vi "Get Path to Plugin UI.vi"(8 "error in (no error)":errorcluster, 11 "Plugin Info":T1 {"Node Status"."Monitor Doubles"."4" format="%#_9g"; "Node Status"."Monitor Doubles"."3" format="%#_9g"; "Node Status"."Monitor Doubles"."2" format="%#_9g"; "Node Status"."Monitor Doubles"."1" format="%#_9g"; "Node Status"."Timing Statistics (us)"."Period"."Avg" format="%_6g"}) -> (0 "error out":errorcluster, 3 "Plugin UI Path":path)   [LabVIEW 2021, in "CIF_Manager_UI.lvclass"]
uses:
  CIF_Manager_UI.lvclass
  Typedef/PluginInfo.ctl
  <vilib>/CIF Foundation/CIF Core/CIFCore/Common/Typedef/Version Simple.ctl
  <vilib>/CIF Foundation/CIF Core/CIFCore/Common/Typedef/gRPC Reported Plugin Status.ctl
  <vilib>/CIF Foundation/CIF Core/CIFCore/Common/Typedef/Plugin State.ctl
  <vilib>/CIF Foundation/CIF Core/CIFCore/Common/Typedef/Timing Statistics.ctl
  <vilib>/CIF Foundation/CIF Core/CIFCore/Common/Typedef/Timing Stats Base.ctl
  <vilib>/CIF Foundation/CIF Core/CIFCore/Common/Typedef/FIFO Statistics.ctl
  <vilib>/CIF Foundation/CIF Core/CIFCore/Common/Typedef/Simple Error.ctl
  <vilib>/CIF Foundation/CIF Core/CIFCore/Common/Typedef/Monitor Doubles.ctl
  <vilib>/CIF Foundation/CIF Core/CIFCore/Common/Typedef/Monitor U64.ctl
  <vilib>/CIF Foundation/CIF Core/CIFCore/Common/Typedef/Monitor I64.ctl
  <vilib>/CIF Foundation/CIF Core/CIFUtilities/CIFConfigurationFile/typedef/Location Type.ctl
  <vilib>/CIF Foundation/CIF Core/CIFCore/Common/Typedef/Errors.ctl
  <vilib>/CIF Foundation/CIF Utilities/Errors/Append Error Location.vi
  <vilib>/CIF Foundation/CIF Core/CIFUtilities/CIFConfigurationFile/CIF Configuration File Location.vi
  <vilib>/CIF Foundation/CIF Core/CIFCore/Common/CIFCoreCommon.lvlib
  <vilib>/CIF Foundation/CIF Core/CIFUtilities/CIFConfigurationFile/CIF Configuration File.lvlib
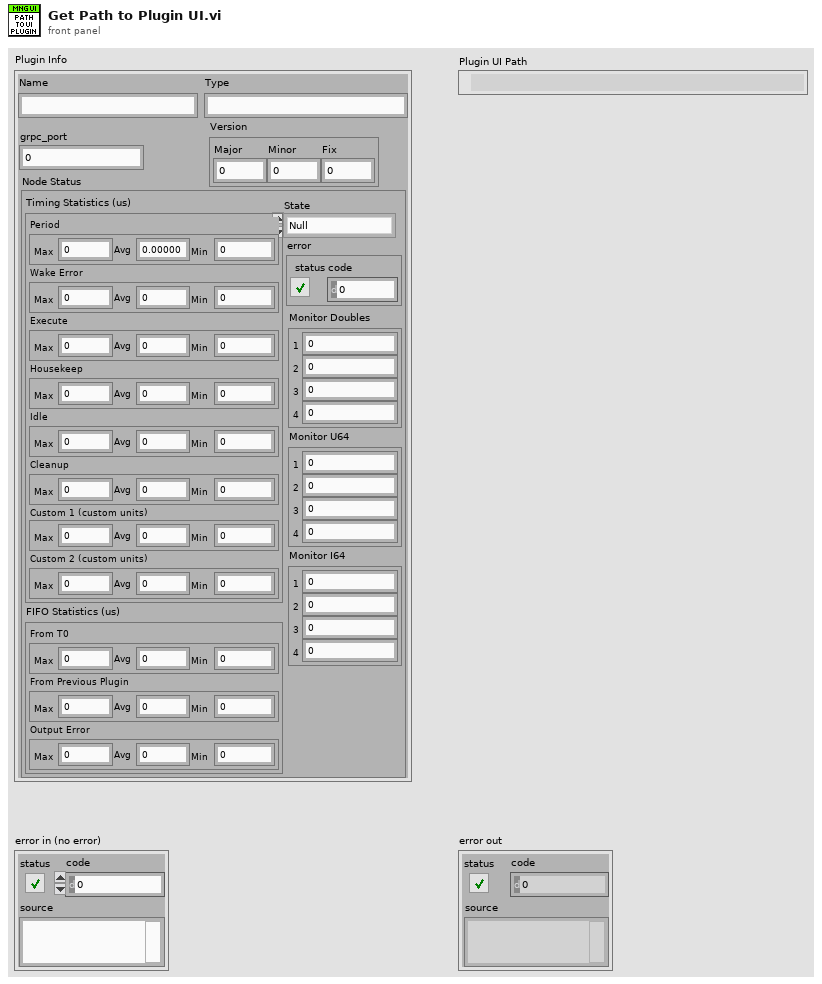
[diagram p1: front panel]
types:
  T1 = typedef "CIF_Manager_UI.lvclass/PluginInfo.ctl" = cluster{"Name":string, "Type":string, "grpc_port":i32, "Version":T2, "Node Status":T3}
  T2 = typedef "CIFCoreCommon.lvlib/Version Simple.ctl" = cluster{"Major":i32, "Minor":i32, "Fix":i32}
  T3 = typedef "CIFCoreCommon.lvlib/gRPC Reported Plugin Status.ctl" = cluster{"State":T4, "Timing Statistics (us)":T5, "FIFO Statistics (us)":T7, "error":T8, "Monitor Doubles":T9, "Monitor U64":T10, "Monitor I64":T11}
  T4 = typedef "CIFCoreCommon.lvlib/Plugin State.ctl" = enum32{"Null", "Creating", "Listening", "Running", "CleaningUp", "Destroying", "Prepared", "FTE_Run"}
  T5 = typedef "CIFCoreCommon.lvlib/Timing Statistics.ctl" = cluster{"Period":T6, "Wake Error":T6, "Execute":T6, "Housekeep":T6, "Idle":T6, "Cleanup":T6, "Custom 1 (custom units)":T6, "Custom 2 (custom units)":T6}
  T6 = typedef "CIFCoreCommon.lvlib/Timing Stats Base.ctl" = cluster{"Max":i64, "Avg":dbl, "Min":i64}
  T7 = typedef "CIFCoreCommon.lvlib/FIFO Statistics.ctl" = cluster{"From T0":T6, "From Previous Plugin":T6, "Output Error":T6}
  T8 = typedef "CIFCoreCommon.lvlib/Simple Error.ctl" = cluster{"status":bool, "code":i32}
  T9 = typedef "CIFCoreCommon.lvlib/Monitor Doubles.ctl" = cluster{"1":dbl, "2":dbl, "3":dbl, "4":dbl}
  T10 = typedef "CIFCoreCommon.lvlib/Monitor U64.ctl" = cluster{"1":u64, "2":u64, "3":u64, "4":u64}
  T11 = typedef "CIFCoreCommon.lvlib/Monitor I64.ctl" = cluster{"1":i64, "2":i64, "3":i64, "4":i64}
  T12 = typedef "CIF Configuration File.lvlib/Location Type.ctl" = enum16{"Config File", "Manager", "Protos", "Plugins", "UI Plugins", "Logs", "Orchestrations", "Loaders"}
  T13 = typedef "CIFCoreCommon.lvlib/Errors.ctl" = enum16{"Invalid Clock ID", "Long Sleep", "gRPC Server Not Found", "Config Parse", "Timestamp Wrap", "Delayed Execution", "Duplicate Channel", "Missing Channel", "Incorrect Type", "Flatten Error", "Unflatten Data", "Unique Name", "Plugin Not Found", "Plugin Type Not Found", "Plugin Version Not Found", "Manager Not Found", "Numerical Issue", "Time Jump", "Clock ID Match", "Channel Length", "Plugin Connection", "gRPC Server Connection", "PPL Name Match", "Build", "Config Log Parse", "Plugin Load", "UI Subpanel Load", "Python Name", "Invalid Name", "Unable to Change Ch Buffer", "Failed Kill", "Failed SysExec", "Function Not Implemented", "Load Timeout", "Invalid FTE"}
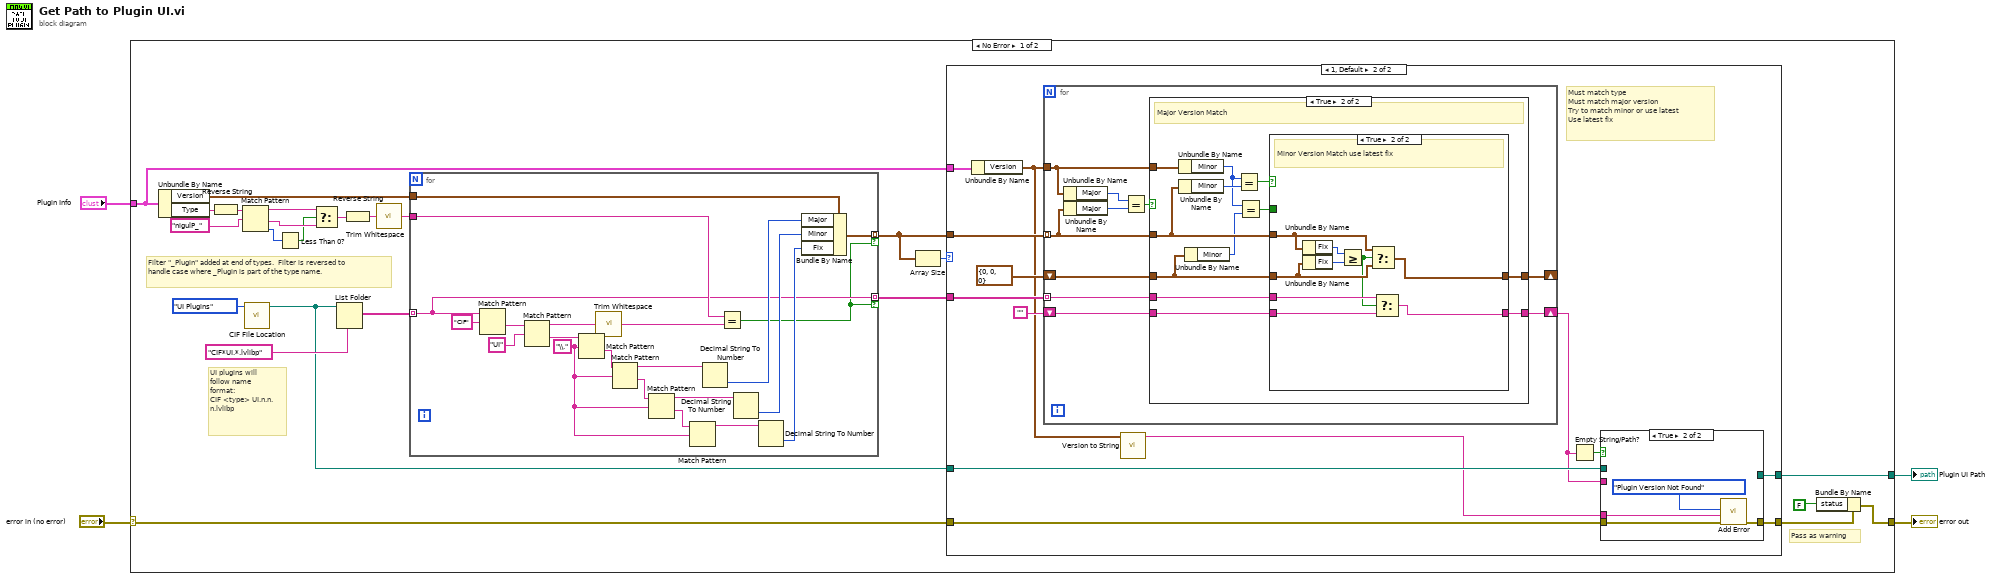
[diagram p0: block diagram]
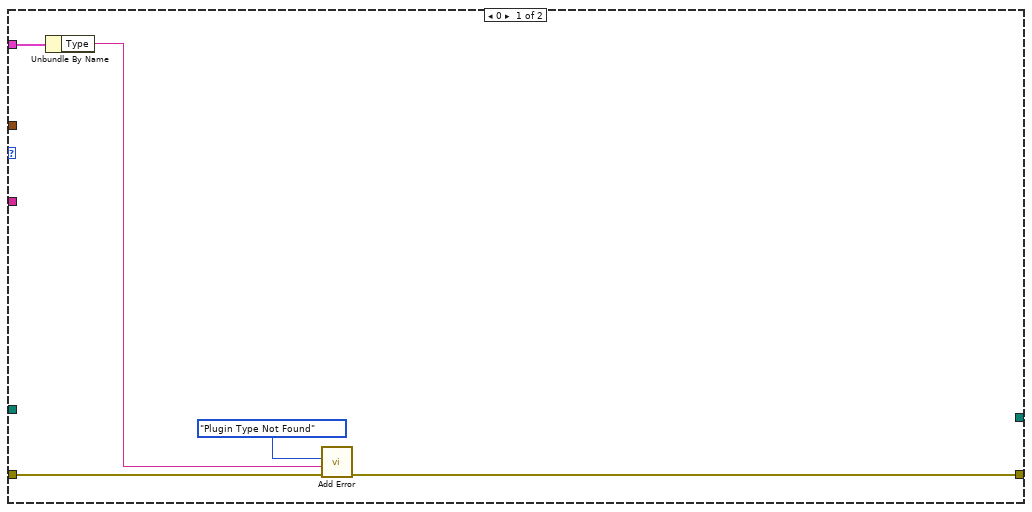
[diagram p2: hidden frame]
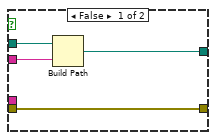
[diagram p3: hidden frame]
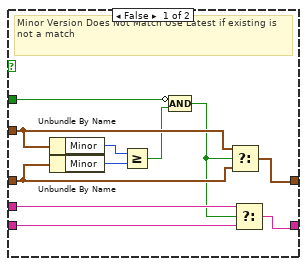
[diagram p5: hidden frame]
diagram:
  n1 = case shown="No Error" "error in (no error)" {
    selector: "error in (no error)" -> [w19 w120]
    tunnel: "Plugin Info" -> [w23 _]
    tunnel: [w16 w120] -> w3
    tunnel: [w20 _] -> w2
    frame No Error {
      # "Filter \"_Plugin\" added at end of types.  Filter is reversed to handle case where _Plugin is part of the type name."
      # "Pass as warning"
      # "UI plugins will follow name format:\nCIF <type> UI.n.n.n.lvlibp"
      n2 = Unbundle By Name(w23) -> ("Version"=w27:T2, "Type"=w14:string)
      n3 = Reverse String(1:w14) -> (0:w13:string)
      n4 = Match Pattern(string=w13, regular expression="nigulP_") -> (before substring=w11:string, after substring=w9:string, offset past match=w8:i32)  [unwired: 1 in, 1 out]
      n5 = call <vilib>:"CIF File Location.vi"("LocationType"=Location_Type."UI Plugins") -> ("Location"=w5:path)  [unwired: 10 in]
      n6 = Less Than 0?(x=w8) -> (x < 0?=w7:bool)
      n7 = Select(t=w11, s=w7, f=w9) -> (s? t:f=w10:string)
      n8 = List Folder(path=w5, pattern="CIF*UI.*.lvlibp") -> (filenames=w22:string[])  [unwired: 2 in, 3 out]
      n9 = Reverse String(1:w10) -> (0:w12:string)
      n10 = call <vilib>:"Trim Whitespace.vi"("string"=w12) -> ("trimmed string"=w26:string)  [unwired: 1 in]
      n11 = for {
        tunnel: w22 -> [w100] mode=indexing
        tunnel: w26 -> [w107]
        tunnel: w27 -> [w101]
        tunnel: [w102] -> w25 mode=indexing if=w99
        tunnel: [w100] -> w21 mode=indexing if=w99
        w113 = "\\." ("regular expression")
        n12 = Match Pattern(string=w100, regular expression="CIF") -> (after substring=w118:string)  [unwired: 1 in, 3 out]
        n13 = Match Pattern(string=w118, regular expression="UI") -> (before substring=w115:string, after substring=w116:string)  [unwired: 1 in, 2 out]
        n14 = Match Pattern(string=w116, regular expression=w113) -> (after substring=w114:string)  [unwired: 1 in, 3 out]
        n15 = call <vilib>:"Trim Whitespace.vi"("string"=w115) -> ("trimmed string"=w106:string)  [unwired: 1 in]
        n16 = Match Pattern(string=w114, regular expression=w113) -> (before substring=w108:string, after substring=w111:string)  [unwired: 1 in, 2 out]
        n17 = Match Pattern(string=w111, regular expression=w113) -> (before substring=w109:string, after substring=w112:string)  [unwired: 1 in, 2 out]
        n18 = Match Pattern(string=w112, regular expression=w113) -> (before substring=w110:string)  [unwired: 1 in, 3 out]
        n19 = Decimal String To Number(string=w108) -> (number=w105:i32)  [unwired: 2 in, 1 out]
        n20 = Equal?(x=w107, y=w106) -> (x = y?=w99:bool)
        n21 = Decimal String To Number(string=w109) -> (number=w104:i32)  [unwired: 2 in, 1 out]
        n22 = Decimal String To Number(string=w110) -> (number=w103:i32)  [unwired: 2 in, 1 out]
        n23 = Bundle By Name(cluster=w101, "Major"=w105, "Minor"=w104, "Fix"=w103) -> (w102:T2)
      }
      n24 = Array Size(array=w25) -> (size(s)=w24:i32)
      n25 = case shown="1, Default" w24 {
        tunnel: w25 -> [_ w46]
        tunnel: w19 -> [w32 w37]
        tunnel: w23 -> [w33 w45]
        tunnel: [w31 w36] -> w17
        tunnel: w21 -> [_ w43]
        tunnel: w5 -> [_ w42]
        tunnel: [_ w41] -> w20
        frame 0 {
          n26 = Unbundle By Name(w33) -> ("Type"=w30:string)
          n27 = call <vilib>:"Add Error.vi"("error in (no error)"=w32, "String to Append"=w30, "Error"=Errors."Plugin Type Not Found") -> ("error out"=w31:errorcluster)  [unwired: 8 in]
        }
        frame 1, Default {
          # "Must match type\nMust match major version\nTry to match minor or use latest\nUse latest fix"
          n28 = Unbundle By Name(w45) -> ("Version"=w35:T2)
          n29 = for {
            tunnel: w46 -> [w60] mode=indexing
            tunnel: w35 -> [w61]
            shift-right: [w58] -> _
            shift-left: T2 {"Major"=0, "Minor"=0, "Fix"=0} ("Version") -> [w59]
            tunnel: w43 -> [w57] mode=indexing
            shift-right: [w56] -> w39
            shift-left: "" -> [w55]
            n30 = Unbundle By Name(w61) -> ("Major"=w63:i32)
            n31 = Unbundle By Name(w60) -> ("Major"=w64:i32)
            n32 = Equal?(x=w63, y=w64) -> (x = y?=w62:bool)
            n33 = case shown="True" w62 {
              tunnel: w61 -> [_ w76]
              tunnel: w60 -> [_ w75]
              tunnel: w59 -> [w66 w70]
              tunnel: [w66 w74] -> w58
              tunnel: w57 -> [_ w73]
              tunnel: [w65 w72] -> w56
              tunnel: w55 -> [w65 w71]
              frame False {
                # "Major Version Does Not Match"
              }
              frame True {
                # "Major Version Match"
                n34 = Unbundle By Name(w76) -> ("Minor"=w68:i32)
                n35 = Unbundle By Name(w75) -> ("Minor"=w78:i32)
                n36 = Unbundle By Name(w70) -> ("Minor"=w69:i32)
                n37 = Equal?(x=w68, y=w78) -> (x = y?=w77:bool)
                n38 = Equal?(x=w68, y=w69) -> (x = y?=w67:bool)
                n39 = case shown="True" w77 {
                  tunnel: w75 -> [w89 w98]
                  tunnel: w70 -> [w88 w97]
                  tunnel: [w85 w96] -> w74
                  tunnel: w73 -> [w84 w95]
                  tunnel: [w82 w94] -> w72
                  tunnel: w71 -> [w83 w93]
                  tunnel: w67 -> [w80 _]
                  frame False {
                    # "Minor Version Does Not Match Use Latest if existing is not a match"
                    n40 = Unbundle By Name(w89) -> ("Minor"=w87:i32)
                    n41 = Unbundle By Name(w88) -> ("Minor"=w86:i32)
                    n42 = Greater Or Equal?(x=w87, y=w86) -> (x >= y?=w81:bool)
                    n43 = Compound Arithmetic op=AND(invert w80, w81) -> (w79:bool)
                    n44 = Select(t=w89, s=w79, f=w88) -> (s? t:f=w85:T2)
                    n45 = Select(t=w84, s=w79, f=w83) -> (s? t:f=w82:string)
                  }
                  frame True {
                    # "Minor Version Match use latest fix"
                    n46 = Unbundle By Name(w98) -> ("Fix"=w92:i32)
                    n47 = Unbundle By Name(w97) -> ("Fix"=w91:i32)
                    n48 = Greater Or Equal?(x=w92, y=w91) -> (x >= y?=w90:bool)
                    n49 = Select(t=w98, s=w90, f=w97) -> (s? t:f=w96:T2)
                    n50 = Select(t=w95, s=w90, f=w93) -> (s? t:f=w94:string)
                  }
                }
              }
            }
          }
          n51 = call <vilib>:"Version to String.vi"("Version"=w35) -> ("Version String"=w34:string)  [unwired: 10 in]
          n52 = Empty String/Path?(string/path=w39) -> (empty?=w38:bool)
          n53 = case shown="True" w38 {
            tunnel: w42 -> [w50 _]
            tunnel: w39 -> [w49 _]
            tunnel: [w48 _] -> w41
            tunnel: w37 -> [w47 w53]
            tunnel: [w47 w54] -> w36
            tunnel: w34 -> [_ w52]
            frame False {
              n54 = Build Path(base path=w50, name or relative path=w49) -> (appended path=w48:path)
            }
            frame True {
              n55 = call <vilib>:"Add Error.vi"("error in (no error)"=w53, "String to Append"=w52, "Error"=Errors."Plugin Version Not Found") -> ("error out"=w54:errorcluster)  [unwired: 8 in]
            }
          }
        }
      }
      n56 = Bundle By Name(cluster=w17, "status"=FALSE) -> (w16:errorcluster)
    }
    frame Error {
    }
  }
  "error out" <- w3
  "Plugin UI Path" <- w2
